vi "Read Dev.Modules.vi"(8 "error in (no error)":errorcluster, 11 "SLSC Remote in":refnum<class "SLSC Remote.lvclass">) -> (0 "error out":errorcluster, 2 "Dev.Modules":refnum<k21>[](array[refnum]), 3 "SLSC Remote out":refnum<class "SLSC Remote.lvclass">)   [LabVIEW 2015, in "SLSC Remote.lvclass"]
uses:
  SLSC Remote.lvclass
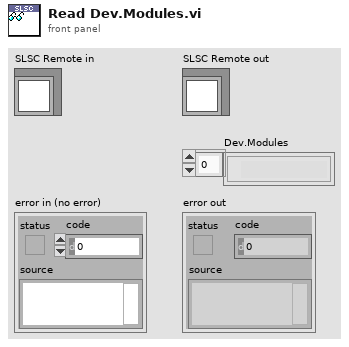
[diagram p1: front panel]
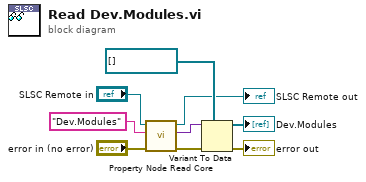
[diagram p0: block diagram]
diagram:
  n1 = call "Property Node Read Core.vi"("error in (no error)"="error in (no error)", "property"="Dev.Modules", "SLSC Remote in"="SLSC Remote in") -> ("error out"=w7:errorcluster, "value"=w8:variant, "SLSC Remote out"=→"SLSC Remote out":refnum<class "SLSC Remote.lvclass">)  [unwired: 6 in]
  n2 = Variant To Data(error in=w7, type=refnum<k21>[] [] ("Dev.Modules"), Variant=w8) -> (data=→"Dev.Modules":refnum<k21>[], error out=→"error out":errorcluster)
